vi "test file IO.vi"() -> ()   [LabVIEW 2017]
uses:
  <vilib>/Utility/file.llb/Read Delimited Spreadsheet (DBL).vi
panel:
  in  "Exp. counter":i32=100
  in  "Experiment file path":path
  in  "Experiment para. file path":path
  out "Number of exp.":i32
  out "Exp. parameters":dbl[][](array[numeric])
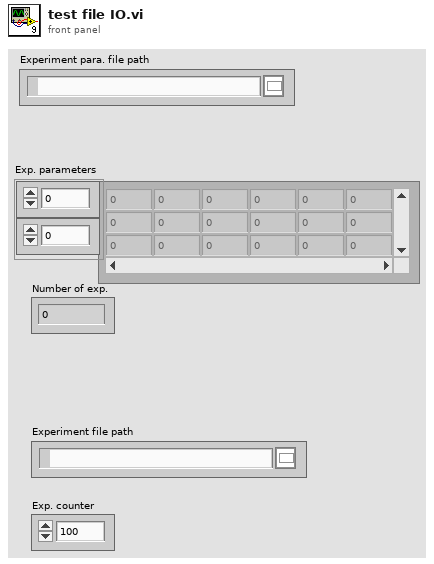
[diagram p1: front panel]
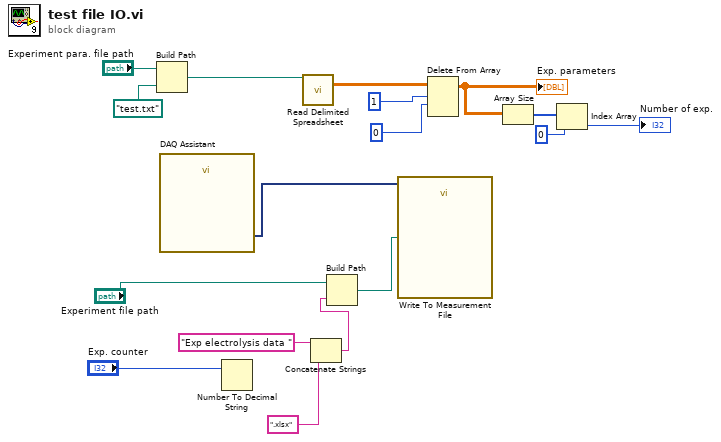
[diagram p0: block diagram]
diagram:
  n1 = Build Path(base path="Experiment para. file path", name or relative path=path "test.txt" ("Experiment para. file path")) -> (appended path=w8:path)
  n2 = call "DAQ Assistant"() -> ("data"=w2:dynamicdata)  [unwired: 17 in, 2 out]
  n3 = Number To Decimal String(number="Exp. counter") -> ()  [unwired: 1 in, 1 out]
  n4 = call-poly <vilib>:"Read Delimited Spreadsheet.vi"("file path (dialog if empty)"=w8) -> ("all rows"=w17:dbl[][])  [unwired: 9 in, 5 out]
  n5 = Concatenate Strings("Exp electrolysis data " ("string"), ".xlsx" ("string")) -> (w6:string)  [unwired: 1 in]
  n6 = Build Path(base path="Experiment file path", name or relative path=w6) -> (appended path=w3:path)
  n7 = call "Write To Measurement File"("Signals"=w2, "Filename"=w3) -> ()  [unwired: 15 in, 3 out]
  n8 = Delete From Array(array=w17, length=1 ("index (row)"), index (row)=0) -> (array with subset deleted=w14:dbl[][])  [unwired: 1 in, 1 out]
  "Exp. parameters" <- w14
  n9 = Array Size(array=w14) -> (size(s)=w13:i32[])
  n10 = Index Array(array=w13, index=0) -> (element=→"Number of exp.":i32)
